vi "get_physical_channel.vi"(8 "error in (no error)":errorcluster, 11 "DAQmxWriteSignals.lvclass in":refnum<class "SignalWriterDL090202DAQmx.lvclass">) -> (0 "error out":errorcluster, 2 "physical channel":tag, 3 "DAQmxWriteSignals.lvclass out":refnum<class "SignalWriterDL090202DAQmx.lvclass">)   [LabVIEW 2010, in "SignalWriterDL090202DAQmx.lvclass"]
uses:
  SignalWriterDL090202DAQmx.lvclass
  SignalWriterDL090202DAQmx.lvclass/SignalWriterDL090202DAQmx.ctl
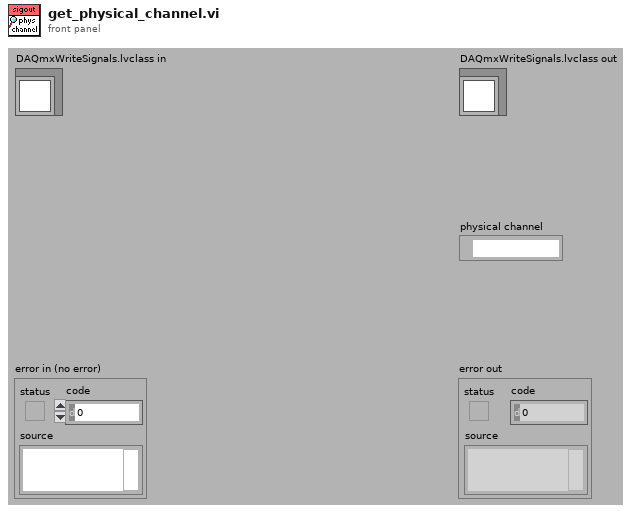
[diagram p1: front panel]
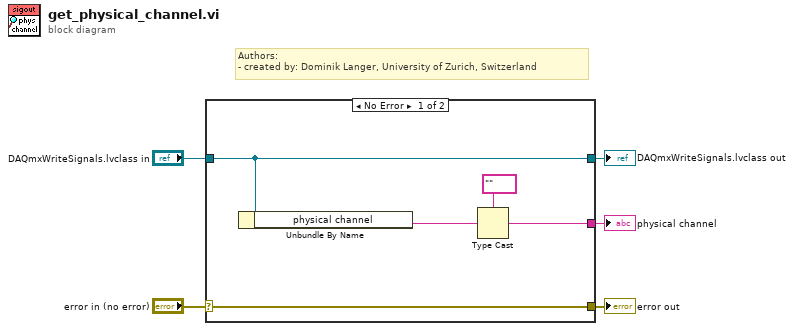
[diagram p0: block diagram]
diagram:
  # "Authors: \n- created by: Dominik Langer, University of Zurich, Switzerland"
  n1 = case shown="No Error" "error in (no error)" {
    selector: "error in (no error)" -> [w10 w11]
    tunnel: [w10 w11] -> w4
    tunnel: [w9 w12] -> w2
    tunnel: "DAQmxWriteSignals.lvclass in" -> [w9 w12]
    tunnel: [w7 _] -> w1
    frame No Error {
      n2 = Unbundle By Name(w9) -> ("physical channel"=w8:string)
      n3 = Type Cast(type=tag "" ("shutter digital output line"), x=w8) -> (*(type *) &x=w7:tag)
    }
    frame Error {
    }
  }
  "error out" <- w4
  "DAQmxWriteSignals.lvclass out" <- w2
  "physical channel" <- w1
